vi "mangle_name.vi"(11 "String in":string) -> (3 "String out":string)   [LabVIEW 2011]
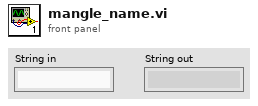
[diagram p1: front panel]
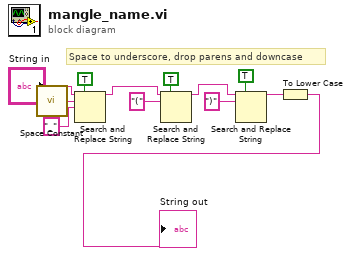
[diagram p0: block diagram]
diagram:
  # "Space to underscore, drop parens and downcase"
  n1 = call <vilib>:"Space Constant.vi"() -> ("String"=w1:string)
  n2 = Search and Replace String(replace all?=TRUE ("replace all? (F)"), input string="String in", search string=w1, replace string="_" ("replace string (\"\")")) -> (result string=w6:string)  [unwired: 4 in, 3 out]
  n3 = Search and Replace String(replace all?=TRUE ("replace all? (F)"), input string=w6, search string="(" ("replace string (\"\")")) -> (result string=w11:string)  [unwired: 5 in, 3 out]
  n4 = Search and Replace String(replace all?=TRUE ("replace all? (F)"), input string=w11, search string=")" ("replace string (\"\")")) -> (result string=w10:string)  [unwired: 5 in, 3 out]
  n5 = To Lower Case(string=w10) -> (all lower case string=→"String out":string)
